vi "DSF.Shared.Configuration.Transfer.From String.vi"(8 "error in (no error)":errorcluster, 10 "String":string) -> (0 "error out":errorcluster, 3 "Transfer Configuration out":refnum<class "DSF.Shared.Configuration.Transfer.lvclass">)   [LabVIEW 2016, in "DSF.Shared.lvlib" / "DSF.Shared.Configuration.Transfer.lvclass"]
uses:
  DSF.Shared.Configuration.Transfer.lvclass
  C:/Git/Sourcetree/DSF/Source/Shared/Classes/Configuration/DSF.Shared.Configuration.lvclass
  Configuration/DSF.Shared.Configuration.lvclass
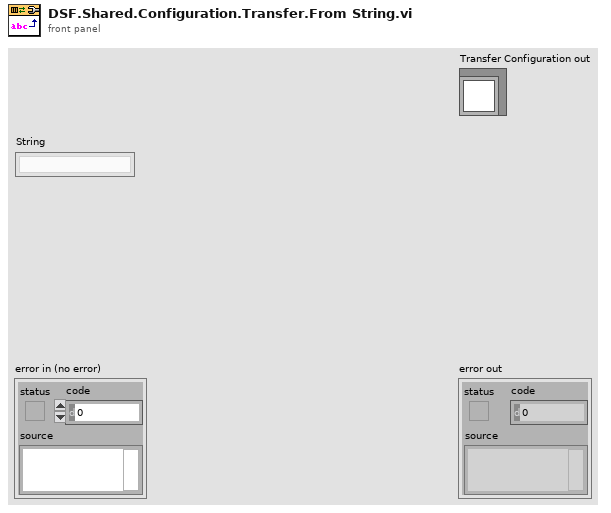
[diagram p1: front panel]
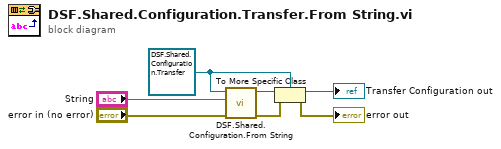
[diagram p0: block diagram]
diagram:
  w5 = refnum<class "DSF.Shared.Configuration.Transfer.lvclass"> refnum ("Transfer Configuration out")
  n1 = call "DSF.Shared.Configuration.From String.vi"("error in (no error)"="error in (no error)", "String"="String", "Configuration in"=w5) -> ("error out"=w3:errorcluster, "Configuration out"=w6:refnum<class "DSF.Shared.Configuration.lvclass">)  [unwired: 7 in]
  n2 = To More Specific Class(target class=w5, reference=w6, error in=w3) -> (specific class reference=→"Transfer Configuration out":refnum<class "DSF.Shared.Configuration.Transfer.lvclass">, error out=→"error out":errorcluster)
